vi "QUERY_TELEM_Channel.vi"(5 "AiP_ele.":i32, 7 "AiP_No.":i32, 8 "error in":errorcluster, 11 "TRXmode":u16(ring)=1 items=["QUERY_TELEM_2 (V)"=2, "QUERY_TELEM_1 (H)"=1]) -> (0 "error out":errorcluster, 3 "pdet":i32)   [LabVIEW 2023, in "Clover_Cell.lvlib"]
uses:
  Clover_Cell.lvlib
panel:
  in  "TCPIPin":T1={"address"="192.168.100.111", "remote port or service name"=5025, "timeout ms (60000)"=10000}
  out "size(s)":i32
  # "CLC_Gen4_L2"
  # "AiP_1 : 0\nAiP_2 : 1\nAiP_3 : 2\nAiP_4 : 3\nAiP_5 : 4\nAiP_6 : 5\nAiP_7 : 6\nAiP_8 : 7"
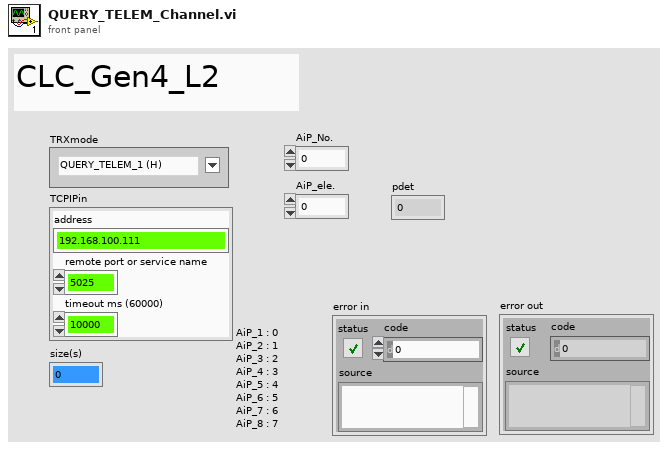
[diagram p1: front panel]
types:
  T1 = cluster{"address":string, "remote port or service name":u16, "timeout ms (60000)":i32}
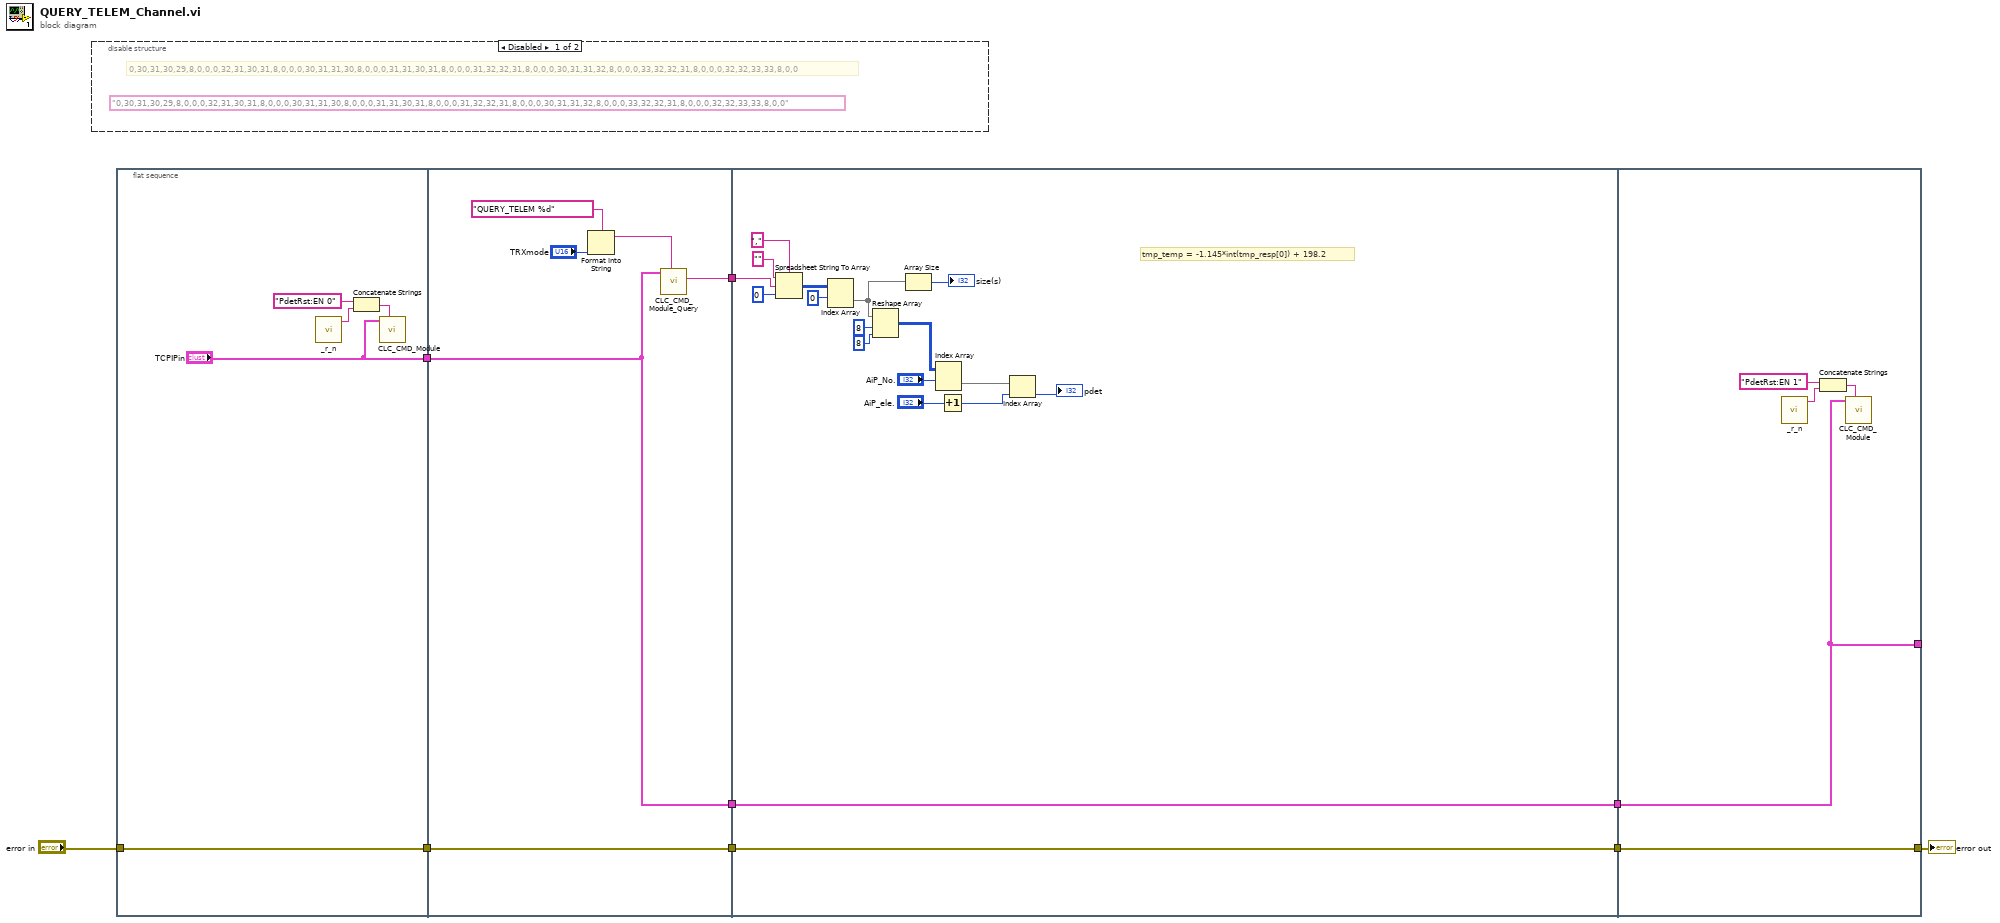
[diagram p0: block diagram]
diagram:
  n1 = disable-structure shown="Disabled" {
    frame Disabled {
      (unwired) "0,30,31,30,29,8,0,0,0,32,31,30,31,8,0,0,0,30,31,31,30,8,0,0,0,31,31,30,31,8,0,0,0,31,32,32,31,8,0,0,0,30,31,31,32,8,0,0,0,33,32,32,31,8,0,0,0,32,32,33,33,8,0,0"
      # "0,30,31,30,29,8,0,0,0,32,31,30,31,8,0,0,0,30,31,31,30,8,0,0,0,31,31,30,31,8,0,0,0,31,32,32,31,8,0,0,0,30,31,31,32,8,0,0,0,33,32,32,31,8,0,0,0,32,32,33,33,8,0,0"
    }
    frame Enabled {
    }
  }
  n2 = flat-sequence {
    tunnel: ["TCPIPin"] -> w7
    tunnel: "error in" -> [w10]
    tunnel: [w10] -> w2
    tunnel: [w20] -> w9
    tunnel: [w16] -> w8
    tunnel: w7 -> [w16]
    tunnel: [w15] -> w3
    tunnel: w2 -> [w15]
    tunnel: w9 -> [w36]
    tunnel: w8 -> [w28]
    tunnel: [w28] -> w6
    tunnel: [w22] -> w4
    tunnel: w3 -> [w22]
    tunnel: [w40] -> _
    tunnel: w6 -> [w40]
    tunnel: [w39] -> w1
    tunnel: w4 -> [w39]
    frame #0 {
      n3 = call "_r_n.vi"() -> ("command"=w13:string)  [unwired: 5 in]
      n4 = Concatenate Strings("PdetRst:EN 0" ("CMD in"), w13) -> (w12:string)
      n5 = call "CLC_CMD_Module.vi"("CMD in"=w12, "TCPIPin"="TCPIPin") -> ()  [unwired: 6 in, 4 out]
    }
    frame #1 {
      n6 = Format Into String(format string="QUERY_TELEM %d" ("data in"), "TRXmode") -> (resulting string=w17:string)  [unwired: 2 in, 1 out]
      n7 = call "CLC_CMD_Module_Query.vi"("CMD in"=w17, "TCPIPin"=w16) -> ("data out"=w20:string)  [unwired: 7 in, 2 out]
    }
    frame #2 {
      # "tmp_temp = -1.145*int(tmp_resp[0]) + 198.2"
      n8 = Spreadsheet String To Array(delimiter (Tab)=",", format string="", spreadsheet string=w36, array type (2D Dbl)=0) -> (array=w32:i32[][])
      n9 = Index Array(array=w32, index (row)=0 ("disabled index (col)")) -> (element=w30:i32[])  [unwired: 1 in]
      n10 = Reshape Array(w30, 8 ("dimension size"), 8 ("dimension size")) -> (w26:i32[][])
      n11 = Array Size(array=w30) -> (size(s)=→"size(s)":i32)
      n12 = Index Array(array=w26, index (row)="AiP_No.") -> (element=w25:i32[])  [unwired: 1 in]
      n13 = Increment(x="AiP_ele.") -> (x+1=w21:i32)
      n14 = Index Array(array=w25, index=w21) -> (element=→"pdet":i32)
    }
    frame #3 {
      n15 = call "_r_n.vi"() -> ("command"=w42:string)  [unwired: 5 in]
      n16 = Concatenate Strings("PdetRst:EN 1" ("CMD in"), w42) -> (w43:string)
      n17 = call "CLC_CMD_Module.vi"("CMD in"=w43, "TCPIPin"=w40) -> ()  [unwired: 6 in, 4 out]
    }
  }
  "error out" <- w1
